vi "Field Draw Field(Quadrada).vi"(5 "FieldRef":refnum<class "Field.lvclass">, 8 "new picture in":picture, 9 "Offset":cluster{"Width":dbl, "Height":dbl}, 10 "Scale":dbl, 11 "Project":T1=enum."VSS") -> (0 "new picture out":picture, 1 "Offset Out":cluster{"Width":dbl, "Height":dbl}, 2 "Scale Out":dbl)   [LabVIEW 2020]
uses:
  Field_class/Field.lvclass
  Parameters_class/Project.ctl
panel:
  in  "left":i16=1
  in  "rect":T2
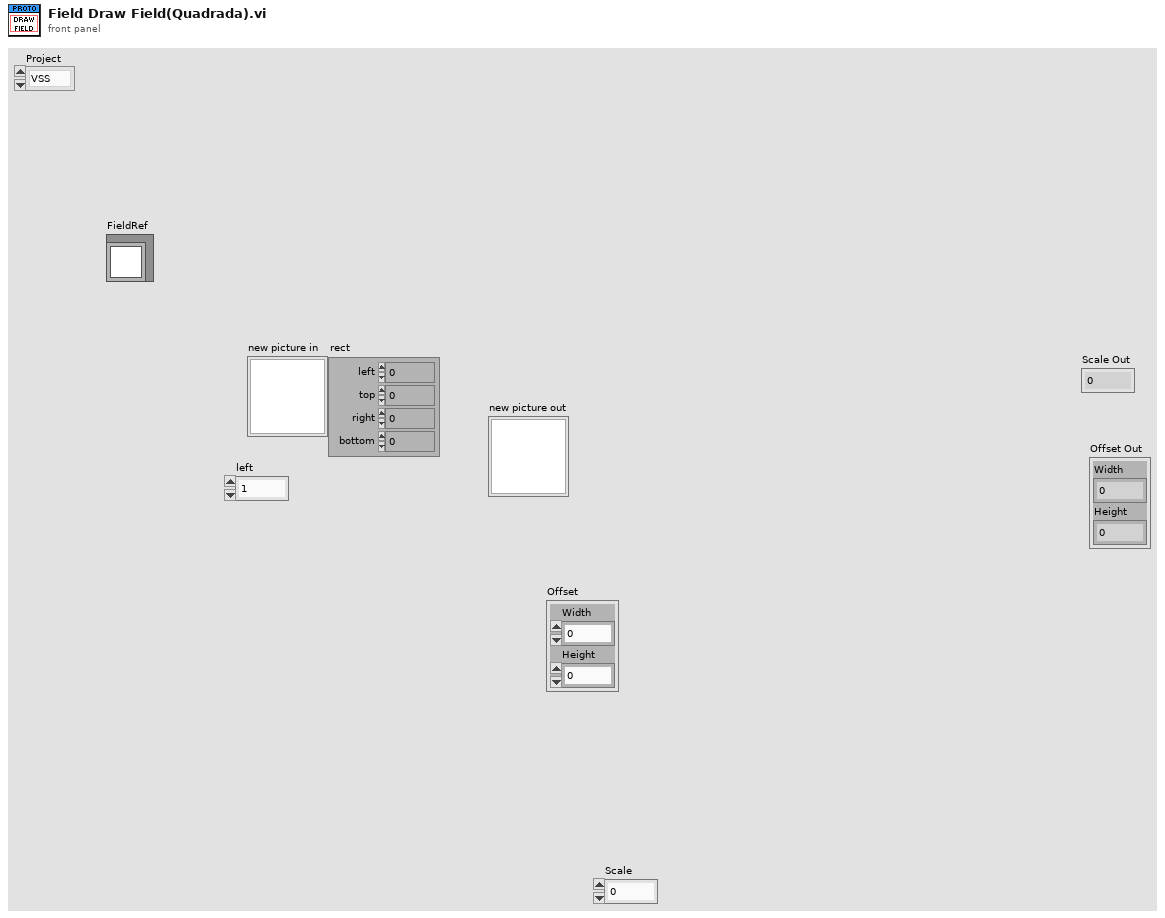
[diagram p1: front panel]
types:
  T1 = typedef "Project.ctl" = enum16{"SSL", "VSS"}
  T2 = cluster{"left":i16, "top":i16, "right":i16, "bottom":i16}
  T3 = cluster{"boundary_width":i32, "center_circle_radius":i32, "defense_stretch":i32, "defense_width_or_radius":i32, "field_length":i32, "field_width":i32, "free_kick_from_defense_dist":i32, "goal_depth":i32, "goal_wall_width":i32, "goal_width":i32, "line_width":i32, "penalty_line_from_spot_dist":i32, "penalty_spot_from_field_line_dist":i32, "referee_width":i32}
  T4 = cluster{"Width":i16, "Style":enum32{"Solid", "Dash", "Dot", "DashDot", "DashDotDot"}}
  T5 = cluster{"boundary_width":dbl, "center_circle_radius":dbl, "defense_stretch":dbl, "defense_width_or_radius":dbl, "field_length":dbl, "field_width":dbl, "free_kick_from_defense_dist":dbl, "goal_depth":dbl, "goal_wall_width":dbl, "goal_width":dbl, "line_width":dbl, "penalty_line_from_spot_dist":dbl, "penalty_spot_from_field_line_dist":dbl, "referee_width":dbl}
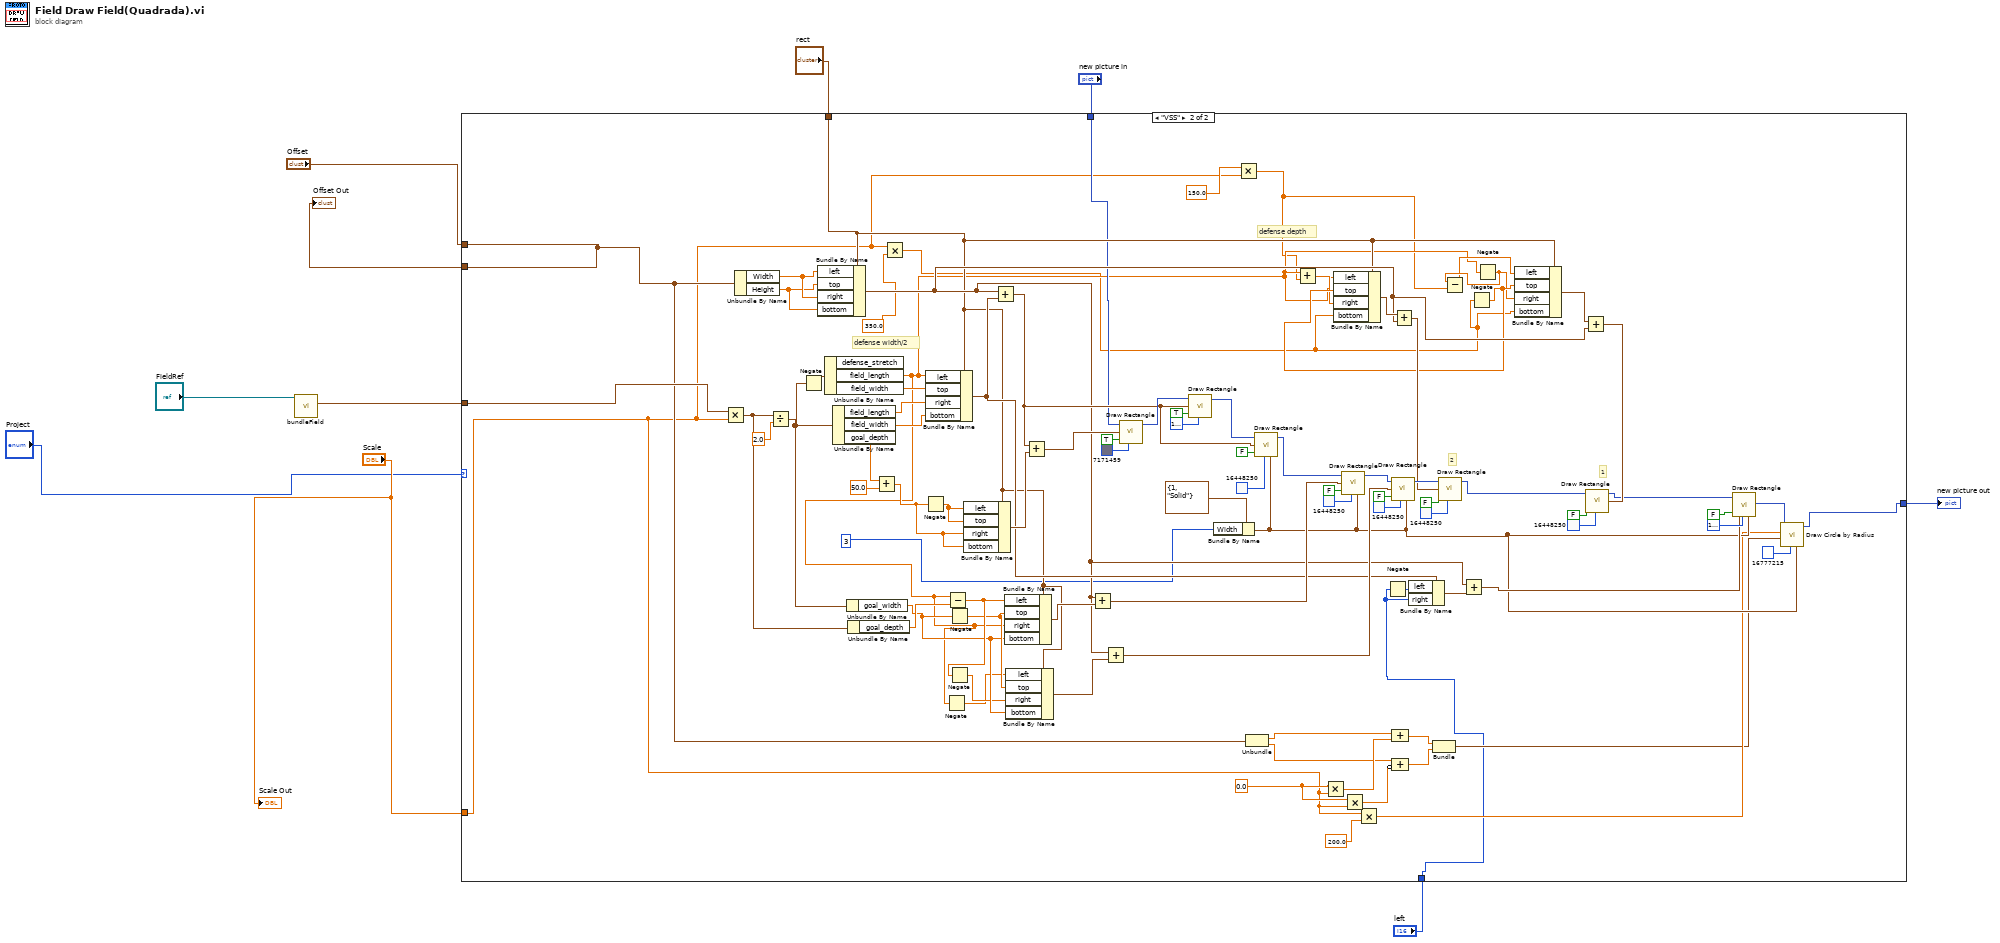
[diagram p0: block diagram]
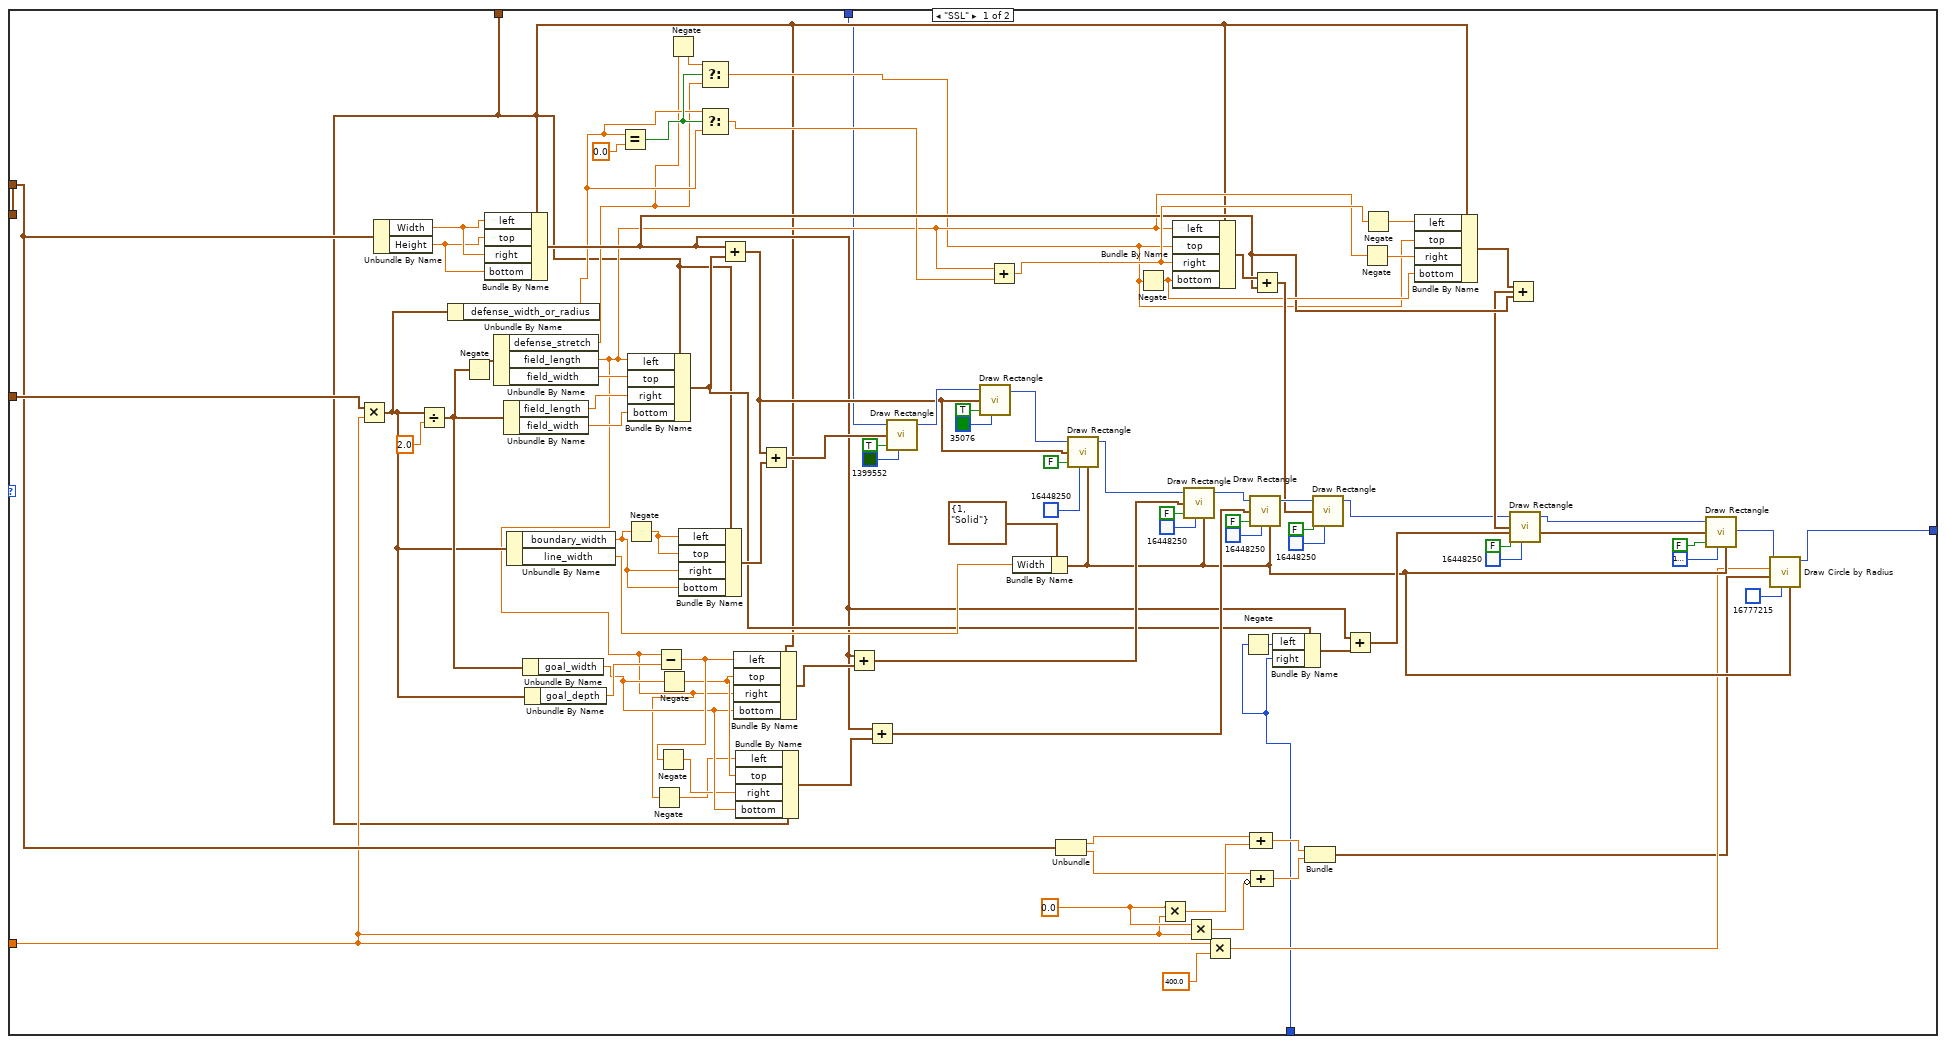
[diagram p2: hidden frame]
diagram:
  n1 = call "bundleField.vi"("Field in"="FieldRef") -> ("Cluster"=w9:T3)  [unwired: 8 in, 2 out]
  n2 = case shown="\"VSS\"" "Project" {
    tunnel: w9 -> [w17 w120]
    tunnel: [w16 w119] -> w8
    tunnel: "Offset" -> [w16 w119]
    tunnel: "Scale" -> [w15 w103]
    tunnel: "rect" -> [w14 w118]
    tunnel: "new picture in" -> [w13 w117]
    tunnel: "left" -> [w12 w116]
    tunnel: [w11 w115] -> w2
    frame "SSL" {
      w43 = 0.0 ("x")
      n3 = Multiply(x=w17, y=w15) -> (x*y=w42:T5)
      n4 = Unbundle By Name(w16) -> ("Width"=w97:dbl, "Height"=w96:dbl)
      n5 = Divide(x=w42, y=2.0) -> (x/y=w73:T5)
      n6 = Unbundle By Name(w42) -> ("defense_width_or_radius"=w19:dbl)
      n7 = Negate(x=w73) -> (-x=w92:T5)
      n8 = Bundle By Name(cluster=w14, "left"=w97, "top"=w96, "right"=w97, "bottom"=w96) -> (w29:T2)
      n9 = Unbundle By Name(w92) -> ("defense_stretch"=w18:dbl, "field_length"=w24:dbl, "field_width"=w95:dbl)
      n10 = Unbundle By Name(w73) -> ("field_length"=w94:dbl, "field_width"=w93:dbl)
      n11 = Unbundle By Name(w42) -> ("boundary_width"=w90:dbl, "line_width"=w80:dbl)
      n12 = Unbundle By Name(w73) -> ("goal_width"=w67:dbl)
      n13 = Unbundle By Name(w42) -> ("goal_depth"=w72:dbl)
      n14 = Equal?(x=w19, y=0.0) -> (x = y?=w26:bool)
      n15 = Negate(x=w90) -> (-x=w91:dbl)
      n16 = Bundle By Name(cluster=w14, "left"=w24, "top"=w95, "right"=w94, "bottom"=w93) -> (w60:T2)
      n17 = Negate(x=w24) -> (-x=w63:dbl)
      n18 = Subtract(x=w24, y=w72) -> (x-y=w69:dbl)
      n19 = Negate(x=w69) -> (-x=w64:dbl)
      n20 = Negate(x=w67) -> (-x=w68:dbl)
      n21 = Negate(x=w18) -> (-x=w22:dbl)
      n22 = Bundle By Name(cluster=w14, "left"=w91, "top"=w91, "right"=w90, "bottom"=w90) -> (w89:T2)
      n23 = Select(t=w22, s=w26, f=w18) -> (s? t:f=w23:dbl)
      n24 = Select(t=w19, s=w26, f=w19) -> (s? t:f=w25:dbl)
      n25 = Add(x=w29, y=w60) -> (x+y=w53:T2)
      n26 = Bundle By Name(cluster=w14, "left"=w69, "top"=w68, "right"=w24, "bottom"=w67) -> (w71:T2)
      n27 = Bundle By Name(cluster=w14, "left"=w63, "top"=w68, "right"=w64, "bottom"=w67) -> (w66:T2)
      n28 = Add(x=w53, y=w89) -> (x+y=w86:T2)
      n29 = Add(x=w29, y=w71) -> (x+y=w70:T2)
      n30 = Add(x=w29, y=w66) -> (x+y=w65:T2)
      n31 = call <vilib>:"Draw Rectangle.vi"("picture"=w13, "rect"=w86, "fill?(F)"=TRUE, "color(black)"=u32 1399552) -> ("new picture"=w85:picture)  [unwired: 5 in]
      n32 = call <vilib>:"Draw Rectangle.vi"("picture"=w85, "rect"=w53, "fill?(F)"=TRUE, "color(black)"=u32 35076) -> ("new picture"=w82:picture)  [unwired: 5 in]
      n33 = Add(x=w24, y=w25) -> (x+y=w35:dbl)
      n34 = Bundle By Name(cluster=T4 {"Width"=1, "Style"=enum."Solid"} ("pen"), "Width"=w80) -> (w54:T4)
      n35 = Unbundle(w16) -> ("Width"=w51:dbl, "Height"=w48:dbl)
      n36 = call <vilib>:"Draw Rectangle.vi"("picture"=w82, "rect"=w53, "fill?(F)"=FALSE, "color(black)"=u32 16448250, "pen"=w54) -> ("new picture"=w77:picture)  [unwired: 4 in]
      n37 = Negate(x=w23) -> (-x=w33:dbl)
      n38 = Multiply(x=w43, y=w15) -> (x*y=w50:dbl)
      n39 = Bundle By Name(cluster=w14, "left"=w24, "top"=w23, "right"=w35, "bottom"=w33) -> (w38:T2)
      n40 = call <vilib>:"Draw Rectangle.vi"("picture"=w77, "rect"=w70, "fill?(F)"=FALSE, "color(black)"=u32 16448250, "pen"=w54) -> ("new picture"=w74:picture)  [unwired: 4 in]
      n41 = Multiply(x=w43, y=w15) -> (x*y=w47:dbl)
      n42 = Multiply(x=w15, y=sgl 400.0 ("radius")) -> (x*y=w45:dbl)
      n43 = Negate(x=w12) -> (-x=w57:i16)
      n44 = call <vilib>:"Draw Rectangle.vi"("picture"=w74, "rect"=w65, "fill?(F)"=FALSE, "color(black)"=u32 16448250, "pen"=w54) -> ("new picture"=w39:picture)  [unwired: 4 in]
      n45 = Compound Arithmetic op=ADD(w51, w50) -> (w49:dbl)
      n46 = Compound Arithmetic op=ADD(w48, invert w47) -> (w46:dbl)
      n47 = Add(x=w38, y=w29) -> (x+y=w37:T2)
      n48 = Bundle By Name(cluster=w60, "left"=w57, "right"=w12) -> (w59:T2)
      n49 = Bundle(w49, w46) -> (w44:cluster{dbl, dbl})  [unwired: 1 in]
      n50 = call <vilib>:"Draw Rectangle.vi"("picture"=w39, "rect"=w37, "fill?(F)"=FALSE, "color(black)"=u32 16448250) -> ("new picture"=w21:picture)  [unwired: 5 in]
      n51 = Add(x=w29, y=w59) -> (x+y=w58:T2)
      n52 = Negate(x=w24) -> (-x=w36:dbl)
      n53 = Negate(x=w35) -> (-x=w34:dbl)
      n54 = Bundle By Name(cluster=w14, "left"=w34, "top"=w23, "right"=w36, "bottom"=w33) -> (w30:T2)
      n55 = Add(x=w30, y=w29) -> (x+y=w28:T2)
      n56 = call <vilib>:"Draw Rectangle.vi"("picture"=w21, "rect"=w28, "fill?(F)"=FALSE, "color(black)"=u32 16448250) -> ("new picture"=w20:picture)  [unwired: 5 in]
      n57 = call <vilib>:"Draw Rectangle.vi"("picture"=w20, "rect"=w58, "fill?(F)"=FALSE, "color(black)"=u32 16777226, "pen"=w54) -> ("new picture"=w56:picture)  [unwired: 4 in]
      n58 = call <vilib>:"Draw Circle by Radius.vi"("pen"=w54, "color(black)"=u32 16777215, "pixel center"=w44, "radius"=w45, "picture"=w56) -> ("new picture"=w11:picture)  [unwired: 6 in]
    }
    frame "VSS" {
      w134 = 0.0 ("x")
      # "defense width/2"
      # "defense depth"
      # "1"
      # "2"
      n59 = Multiply(x=w120, y=w103) -> (x*y=w133:T5)
      n60 = Unbundle By Name(w119) -> ("Width"=w186:dbl, "Height"=w185:dbl)
      n61 = Divide(x=w133, y=2.0) -> (x/y=w164:T5)
      n62 = Negate(x=w164) -> (-x=w181:T5)
      n63 = Bundle By Name(cluster=w118, "left"=w186, "top"=w185, "right"=w186, "bottom"=w185) -> (w124:T2)
      n64 = Unbundle By Name(w181) -> ("field_length"=w106:dbl, "field_width"=w184:dbl)  [unwired: 1 out]
      n65 = Unbundle By Name(w164) -> ("field_length"=w183:dbl, "field_width"=w182:dbl, "goal_depth"=w113:dbl)
      n66 = Unbundle By Name(w164) -> ("goal_width"=w158:dbl)
      n67 = Unbundle By Name(w133) -> ("goal_depth"=w163:dbl)
      n68 = Add(x=w113, y=50.0) -> (x+y=w112:dbl)
      n69 = Multiply(x=w103, y=350.0) -> (x*y=w102:dbl)
      n70 = Negate(x=w112) -> (-x=w180:dbl)
      n71 = Bundle By Name(cluster=w118, "left"=w106, "top"=w184, "right"=w183, "bottom"=w182) -> (w151:T2)
      n72 = Negate(x=w106) -> (-x=w154:dbl)
      n73 = Subtract(x=w106, y=w163) -> (x-y=w160:dbl)
      n74 = Negate(x=w160) -> (-x=w155:dbl)
      n75 = Negate(x=w158) -> (-x=w159:dbl)
      n76 = Bundle By Name(cluster=w118, "left"=w180, "top"=w180, "right"=w112, "bottom"=w112) -> (w179:T2)
      n77 = Add(x=w124, y=w151) -> (x+y=w144:T2)
      n78 = Bundle By Name(cluster=w118, "left"=w160, "top"=w159, "right"=w106, "bottom"=w158) -> (w162:T2)
      n79 = Bundle By Name(cluster=w118, "left"=w154, "top"=w159, "right"=w155, "bottom"=w158) -> (w157:T2)
      n80 = Add(x=w144, y=w179) -> (x+y=w176:T2)
      n81 = Add(x=w124, y=w162) -> (x+y=w161:T2)
      n82 = Add(x=w124, y=w157) -> (x+y=w156:T2)
      n83 = call <vilib>:"Draw Rectangle.vi"("picture"=w117, "rect"=w176, "fill?(F)"=TRUE, "color(black)"=u32 7171459) -> ("new picture"=w175:picture)  [unwired: 5 in]
      n84 = call <vilib>:"Draw Rectangle.vi"("picture"=w175, "rect"=w144, "fill?(F)"=TRUE, "color(black)"=u32 16777222) -> ("new picture"=w172:picture)  [unwired: 5 in]
      n85 = Bundle By Name(cluster=T4 {"Width"=1, "Style"=enum."Solid"} ("pen"), "Width"=i16 3) -> (w145:T4)
      n86 = Multiply(x=150.0, y=w103) -> (x*y=w101:dbl)
      n87 = Unbundle(w119) -> ("Width"=w142:dbl, "Height"=w139:dbl)
      n88 = call <vilib>:"Draw Rectangle.vi"("picture"=w172, "rect"=w144, "fill?(F)"=FALSE, "color(black)"=u32 16448250, "pen"=w145) -> ("new picture"=w168:picture)  [unwired: 4 in]
      n89 = Add(x=w106, y=w101) -> (x+y=w107:dbl)
      n90 = Multiply(x=w134, y=w103) -> (x*y=w141:dbl)
      n91 = call <vilib>:"Draw Rectangle.vi"("picture"=w168, "rect"=w161, "fill?(F)"=FALSE, "color(black)"=u32 16448250, "pen"=w145) -> ("new picture"=w165:picture)  [unwired: 4 in]
      n92 = Multiply(x=w134, y=w103) -> (x*y=w138:dbl)
      n93 = Multiply(x=w103, y=sgl 200.0 ("radius")) -> (x*y=w136:dbl)
      n94 = Negate(x=w116) -> (-x=w148:i16)
      n95 = call <vilib>:"Draw Rectangle.vi"("picture"=w165, "rect"=w156, "fill?(F)"=FALSE, "color(black)"=u32 16448250, "pen"=w145) -> ("new picture"=w130:picture)  [unwired: 4 in]
      n96 = Compound Arithmetic op=ADD(w142, w141) -> (w140:dbl)
      n97 = Compound Arithmetic op=ADD(w139, invert w138) -> (w137:dbl)
      n98 = Bundle By Name(cluster=w151, "left"=w148, "right"=w116) -> (w150:T2)
      n99 = Bundle(w140, w137) -> (w135:cluster{dbl, dbl})  [unwired: 1 in]
      n100 = Add(x=w124, y=w150) -> (x+y=w149:T2)
      n101 = Negate(x=w102) -> (-x=w110:dbl)
      n102 = Bundle By Name(cluster=w118, "left"=w106, "top"=w110, "right"=w107, "bottom"=w102) -> (w129:T2)
      n103 = Add(x=w129, y=w124) -> (x+y=w128:T2)
      n104 = call <vilib>:"Draw Rectangle.vi"("picture"=w130, "rect"=w128, "fill?(F)"=FALSE, "color(black)"=u32 16448250) -> ("new picture"=w122:picture)  [unwired: 5 in]
      n105 = Negate(x=w106) -> (-x=w109:dbl)
      n106 = Subtract(x=w109, y=w101) -> (x-y=w108:dbl)
      n107 = Bundle By Name(cluster=w118, "left"=w108, "top"=w110, "right"=w109, "bottom"=w102) -> (w125:T2)
      n108 = Add(x=w125, y=w124) -> (x+y=w123:T2)
      n109 = call <vilib>:"Draw Rectangle.vi"("picture"=w122, "rect"=w123, "fill?(F)"=FALSE, "color(black)"=u32 16448250) -> ("new picture"=w121:picture)  [unwired: 5 in]
      n110 = call <vilib>:"Draw Rectangle.vi"("picture"=w121, "rect"=w149, "fill?(F)"=FALSE, "color(black)"=u32 16777226, "pen"=w145) -> ("new picture"=w147:picture)  [unwired: 4 in]
      n111 = call <vilib>:"Draw Circle by Radius.vi"("pen"=w145, "color(black)"=u32 16777215, "pixel center"=w135, "radius"=w136, "picture"=w147) -> ("new picture"=w115:picture)  [unwired: 6 in]
    }
  }
  "Offset Out" <- w8
  "new picture out" <- w2
  "Scale Out" <- "Scale"
